vi "GetGXMLCfgTach.vi"(8 "error in (no error)":errorcluster, 11 "Tachometer in":refnum<class "Tachometer.lvclass">) -> (0 "error out":errorcluster, 2 "TachChanCfg":T1, 3 "Tachometer out":refnum<class "Tachometer.lvclass">)   [LabVIEW 2012, in "Measurement Channels.lvlib" / "Tachometer.lvclass"]
uses:
  Tachometer.lvclass
  TachProps_TD.ctl
  Tachometer.lvclass/Tachometer.ctl
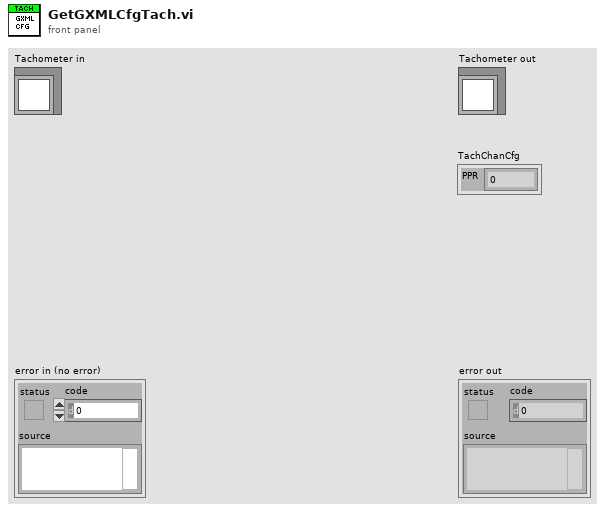
[diagram p1: front panel]
types:
  T1 = typedef "Measurement Channels.lvlib/Tachometer.lvclass/TachProps_TD.ctl" = cluster{"PPR":dbl}
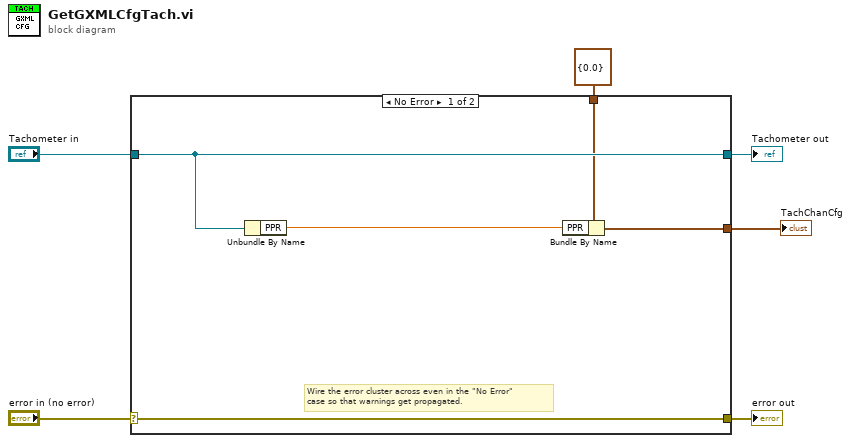
[diagram p0: block diagram]
diagram:
  n1 = case shown="No Error" "error in (no error)" {
    selector: "error in (no error)" -> [w11 w14]
    tunnel: [w11 w14] -> w5
    tunnel: [w10 w13] -> w3
    tunnel: "Tachometer in" -> [w10 w13]
    tunnel: T1 {"PPR"=0.0} ("TachChanCfg") -> [w9 w12]
    tunnel: [w7 w12] -> w1
    frame No Error {
      # "Wire the error cluster across even in the \"No Error\"\ncase so that warnings get propagated."
      n2 = Unbundle By Name(w10) -> ("PPR"=w8:dbl)
      n3 = Bundle By Name(cluster=w9, "PPR"=w8) -> (w7:T1)
    }
    frame Error {
    }
  }
  "error out" <- w5
  "Tachometer out" <- w3
  "TachChanCfg" <- w1
